vi "Waveform Buffer Generation-Current (multi).vi"(0 "task/channels in":refnum<k21>, 1 "Samples per Buffer":dbl=1000.0, 3 "Amplitude":dbl=2.0 format="%0.2p", 5 "Desired Frequency":dbl=1000.0 format="%.2f", 7 "Offset":dbl=0.01 format="%0.2p", 9 "Waveform Type":u16(ring) items=["Sine Wave", "Triangle Wave", "Square Wave", "Sawtooth Wave"], 11 "error in":errorcluster caption="error in (no error)", 12 "Cycles per Buffer":dbl=1.0 format="%.2f") -> (4 "task out":refnum<k21>, 6 "Waveform":waveform(dbl)[](array[waveform]), 10 "Resulting Frequency":dbl format="%.2f", 14 "Resulting Sample Clock Rate":dbl format="%.2f", 15 "error out":errorcluster)   [LabVIEW 2022 SP3]
doc: "This subVI is used to create a Sine, Square, Triangle or Sawtooth Waveform. The inputs to this VI are the Waveform Type, which determines if the output waveform is a Sine, Square, Triangle, or Sawtooth Waveform, the amplitude, Desired Frequency, Samples per Buffer, and Cycles per Buffer. \n\nThe Desired Frequency, Samples per Buffer, and Cycles per Buffer are used to calculate the sample clock rate. The DAQmx Timing property node sets the sample clock rate for the device specified in the task/channels in control. \n\nThe actual, coerced, sample clock rate is returned and used as an input to the Basic Function Generator.vi. The Basic Function Generator returns a waveform of data with timing information.\n\nThe formula below was used to determine the sample clock rate:\n\nDesired Frequency=[(Cycles/Buffer)X(Sample Clock Rate)]/Samples per Buffer\n\nNote: The Block Diagram rearranges the variables to solve for Sample Clock Rate"
uses:
  <vilib>/measure/NI_MABase.lvlib
  <resource>/objmgr/daqmx.rc
panel:
  out "Samples/cycle":dbl format="%0.2f"
  out "Desired Sample Clock Rate":dbl format="%.2f"
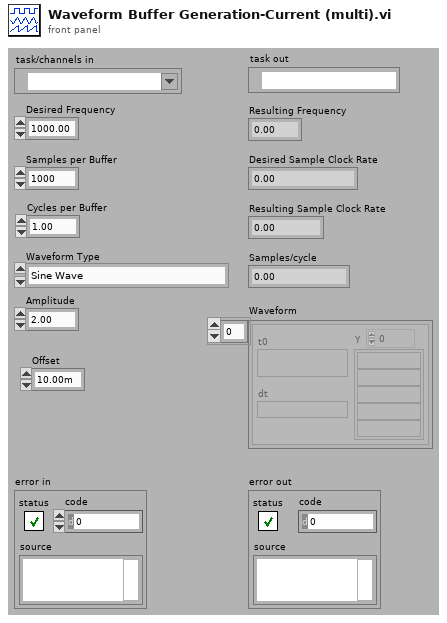
[diagram p1: front panel]
types:
  T1 = cluster{"SampClk.Rate":dbl, "Samples per Buffer":dbl}
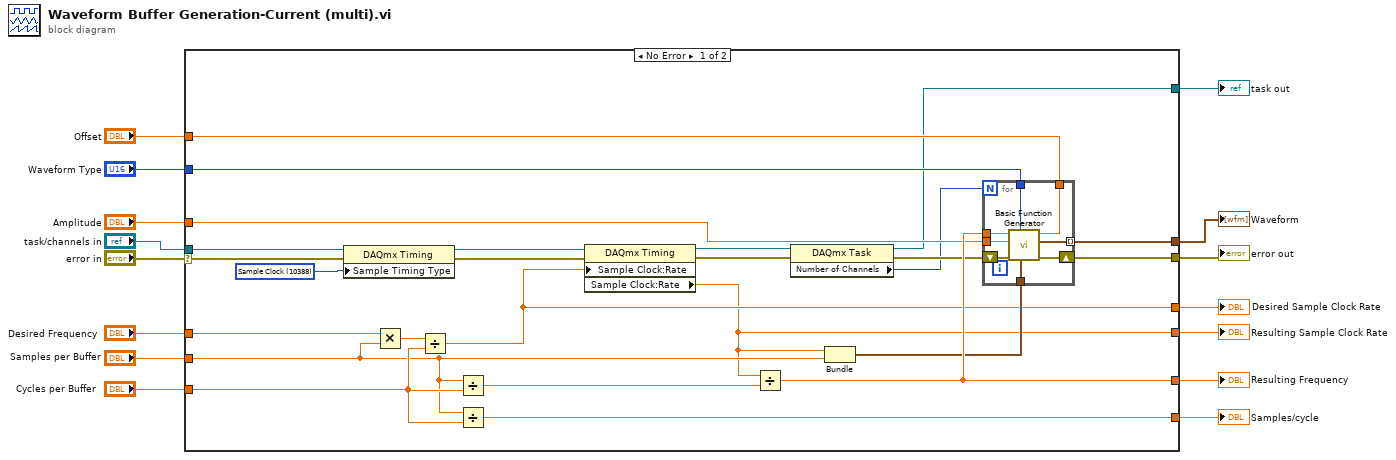
[diagram p0: block diagram]
diagram:
  n1 = case shown="No Error" "error in" {
    selector: "error in" -> [w16 w50]
    tunnel: [w40 _] -> w15
    tunnel: "Desired Frequency" -> [w39 _]
    tunnel: [w36 _] -> w13
    tunnel: "Cycles per Buffer" -> [w35 _]
    tunnel: [w33 _] -> w11
    tunnel: "Waveform Type" -> [w32 _]
    tunnel: "Amplitude" -> [w31 _]
    tunnel: "Samples per Buffer" -> [w30 _]
    tunnel: [w29 _] -> w7
    tunnel: [w28 w50] -> w6
    tunnel: "task/channels in" -> [w24 w49]
    tunnel: "Offset" -> [w23 _]
    tunnel: [w19 w49] -> w3
    tunnel: [w17 _] -> w2
    frame No Error {
      w25 = 10388 items=["Sample Clock"=10388, "Handshake"=10389, "Implicit"=10451, "On Demand"=10390, "Change Detection"=12504] ("SampTimingType")
      n2 = property class="DAQmx Timing"(reference=w24, error in=w16, "Sample Timing Type"=w25) -> (reference out=w27:refnum<k21>, error out=w26:errorcluster)
      n3 = Multiply(x=w39, y=w30) -> (x*y=w37:dbl)
      n4 = Divide(x=w37, y=w35) -> (x/y=w33:dbl)
      n5 = Divide(x=w30, y=w35) -> (x/y=w34:dbl)
      n6 = Divide(x=w30, y=w35) -> (x/y=w36:dbl)
      n7 = property class="DAQmx Timing"(reference=w27, error in=w26, "Sample Clock:Rate"=w33) -> (reference out=w22:refnum<k21>, error out=w21:errorcluster, "Sample Clock:Rate"=w29:dbl)
      n8 = Divide(x=w29, y=w34) -> (x/y=w40:dbl)
      n9 = property class="DAQmx Task"(reference=w22, error in=w21) -> (reference out=w19:refnum<k21>, error out=w20:errorcluster, "Number of Channels"=w18:u32)
      n10 = Bundle("SampClk.Rate"=w29, "Samples per Buffer"=w30) -> (w38:T1)  [unwired: 1 in]
      n11 = for {
        N: w18 -> [_]
        tunnel: w40 -> [w48]
        tunnel: w38 -> [w47]
        tunnel: [w46] -> w17 mode=indexing
        tunnel: w32 -> [w45]
        tunnel: w31 -> [w44]
        tunnel: w23 -> [w42]
        shift-right: [w43] -> w28
        shift-left: w20 -> [w41]
        n12 = call <vilib>:"Basic Function Generator.vi"("offset"=w42, "sampling info"=w47, "signal type"=w45, "error in (no error)"=w41, "amplitude"=w44, "frequency"=w48) -> ("error out"=w43:errorcluster, "signal out"=w46:waveform(dbl))  [unwired: 3 in, 1 out]
      }
    }
    frame Error {
    }
  }
  "Resulting Sample Clock Rate" <- w7
  "Desired Sample Clock Rate" <- w11
  "Resulting Frequency" <- w15
  "Samples/cycle" <- w13
  "error out" <- w6
  "task out" <- w3
  "Waveform" <- w2
